vi "Close.vi"(8 "Error In":errorcluster, 11 "LabVIEWHTTPClient_NET in":refnum<class "HttpClient_NET.lvclass">) -> (0 "Error Out":errorcluster)   [LabVIEW 2018, in "HttpClient_NET.lvlib" / "HttpClient_NET.lvclass"]
uses:
  HttpClient_NET.lvclass
  HttpClient_NET.lvclass/HttpClient_NET.ctl
  System.Net.Http
  Accessors/Read NET_HttpClient.vi
  Accessors/Read NET_HttpClientHandler.vi
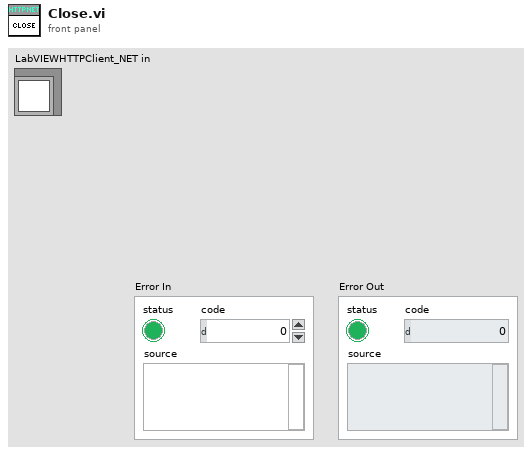
[diagram p1: front panel]
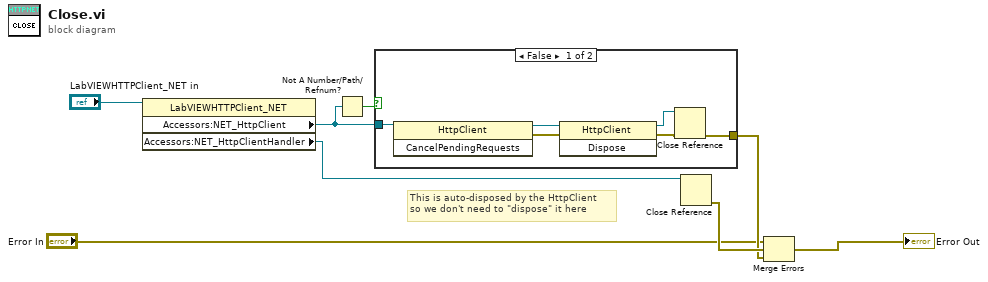
[diagram p0: block diagram]
diagram:
  # "This is auto-disposed by the HttpClient\nso we don't need to \"dispose\" it here"
  n1 = property class="LabVIEWHTTPClient_NET"(reference="LabVIEWHTTPClient_NET in") -> ("Accessors:NET_HttpClient"=w4:refnum<k24>, "Accessors:NET_HttpClientHandler"=w7:refnum<k24>)  [unwired: 1 in, 2 out]
  n2 = Not A Number/Path/Refnum?(number/path/refnum=w4) -> (NaN/Path/Refnum?=w3:bool)
  n3 = case shown="False" w3 {
    tunnel: [w10 _] -> w5
    tunnel: w4 -> [w9 _]
    frame False {
      n4 = invoke class="HttpClient" method="CancelPendingRequests"(reference=w9) -> (reference out=w11:refnum<k24>, error out=w14:errorcluster)  [unwired: 2 in, 1 out]
      n5 = invoke class="HttpClient" method="Dispose"(reference=w11, error in=w14) -> (reference out=w12:refnum<k24>, error out=w13:errorcluster)  [unwired: 1 in, 1 out]
      n6 = Close Reference(reference=w12, error in (no error)=w13) -> (error out=w10:errorcluster)
    }
    frame True {
    }
  }
  n7 = Close Reference(reference=w7) -> (error out=w6:errorcluster)  [unwired: 1 in]
  n8 = Merge Errors("Error In", w6, w5) -> (→"Error Out":errorcluster)
